vi "TestVI.vi"() -> ()   [LabVIEW 2011]
panel:
  out "output 2":i32
  out "output 1":string
  in  "String":string
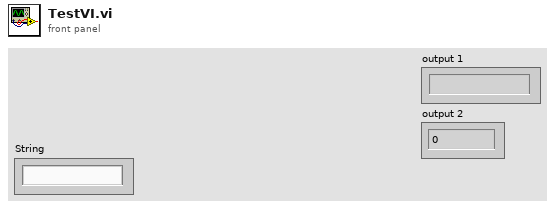
[diagram p1: front panel]
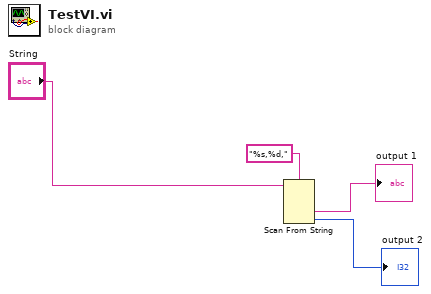
[diagram p0: block diagram]
diagram:
  n1 = Scan From String(format string="%s,%d,", input string="String") -> (output 1=→"output 1":string, output 2=→"output 2":i32)  [unwired: 4 in, 3 out]
